vi "Insert to DB Msg.vi"(8 "error in (no error)":errorcluster, 11 "UI Queue in":refnum<queue>) -> (0 "error out":errorcluster, 3 "UI Queue out":refnum<queue>)   [LabVIEW 2018, in "Message Queue.lvlib"]
uses:
  Message Queue.lvlib
  Message Cluster.ctl
  Enqueue Message (Single).vi
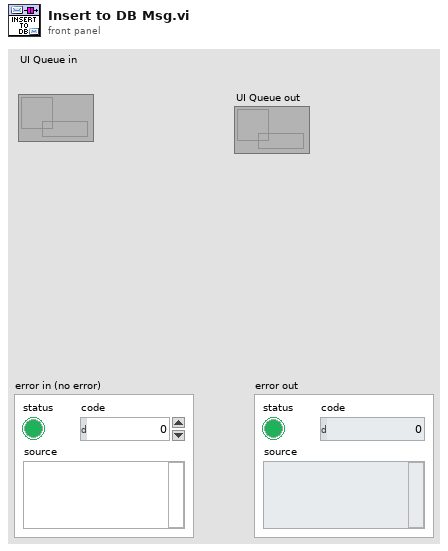
[diagram p1: front panel]
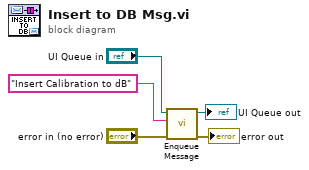
[diagram p0: block diagram]
diagram:
  n1 = call-poly "Enqueue Message.vi"("error in (no error)"="error in (no error)", "Message"="Insert Calibration to dB", "Message Queue"="UI Queue in") -> ("error out"=→"error out":errorcluster, "dup Message Queue"=→"UI Queue out":refnum<queue>)  [unwired: 7 in]
